vi "Post-Run.vi"(8 "error in":errorcluster) -> (0 "error out":errorcluster)   [LabVIEW 2017, in "Controller.lvlib"]
uses:
  Controller.lvlib
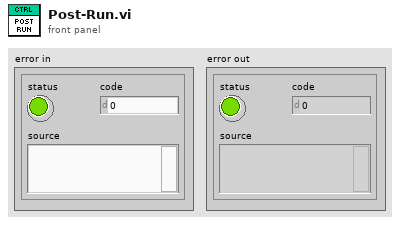
[diagram p1: front panel]
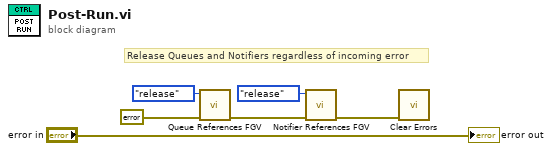
[diagram p0: block diagram]
diagram:
  # "Release Queues and Notifiers regardless of incoming error"
  n1 = call "Queue References FGV.vi"("error in"=errorcluster {"status"=FALSE, "code"=0, "source"=""}, "function"=enum16{"obtain", "get", "release"}."release") -> ("error out"=w4:errorcluster)  [unwired: 8 in, 1 out]
  n2 = call "Notifier References FGV.vi"("error in"=w4, "function"=enum16{"obtain", "get", "release"}."release") -> ("error out"=w3:errorcluster)  [unwired: 8 in, 1 out]
  n3 = call <vilib>:"Clear Errors.vi"("error in (no error)"=w3) -> ()  [unwired: 5 in, 2 out]
  "error out" <- "error in"
